vi "Read File Path.vi"(8 "error in (no error)":errorcluster, 11 "Parameter Generic File in":refnum<class "Parameter Generic File.lvclass">) -> (0 "error out":errorcluster, 2 "File Path":path, 3 "Parameter Generic File out":refnum<class "Parameter Generic File.lvclass">)   [LabVIEW 2019, in "CD Parameter Manager API.lvlib" / "Parameter Generic File.lvclass"]
uses:
  Parameter Generic File.lvclass
  Parameter Generic File.lvclass/Parameter Generic File.ctl
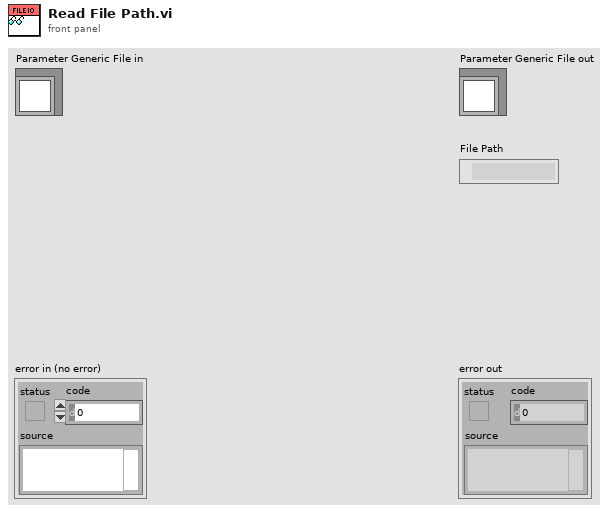
[diagram p1: front panel]
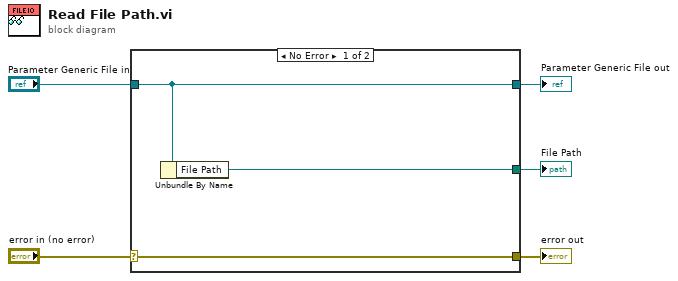
[diagram p0: block diagram]
diagram:
  n1 = case shown="No Error" "error in (no error)" {
    selector: "error in (no error)" -> [w8 w9]
    tunnel: [w8 w9] -> w4
    tunnel: [w7 w10] -> w2
    tunnel: "Parameter Generic File in" -> [w7 w10]
    tunnel: [w6 _] -> w1
    frame No Error {
      n2 = Unbundle By Name(w7) -> ("File Path"=w6:path)
    }
    frame Error {
    }
  }
  "error out" <- w4
  "Parameter Generic File out" <- w2
  "File Path" <- w1
